vi "booleanvisibility.vi"() -> ()   [LabVIEW 2018]
panel:
  in  "stop 3":bool
  in  "String 2":string
  out "Numeric":i32
  in  "Boolean":bool
  in  "stop 2":bool
  in  "String":string
  in  "Boolean 2":bool
  in  "stop":bool
  in  "visible":bool
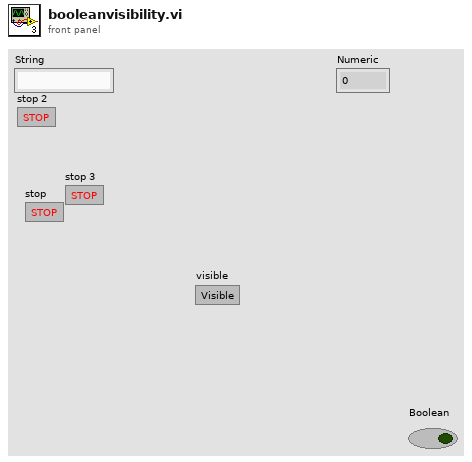
[diagram p1: front panel]
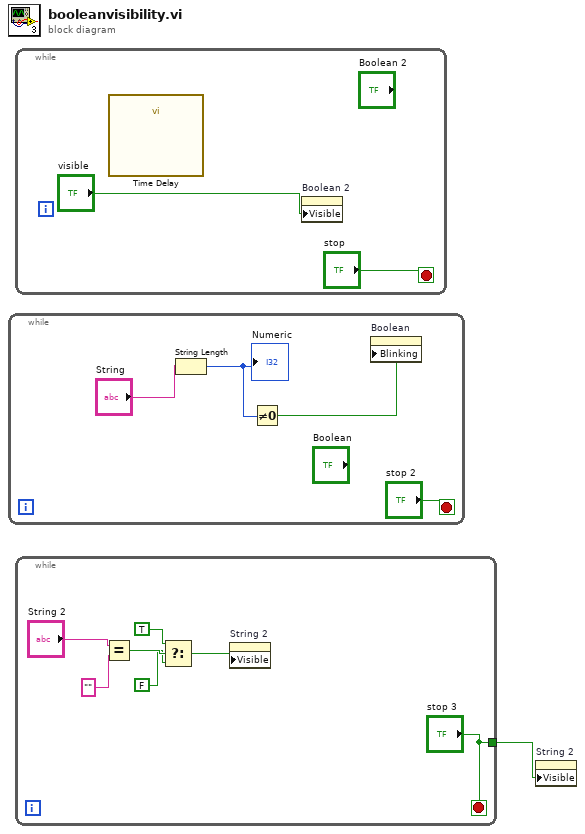
[diagram p0: block diagram]
diagram:
  n1 = while {
    stop <- "stop 2" stop-if-true
    n2 = String Length(string="String") -> (length=w3:i32)
    "Numeric" <- w3
    n3 = Not Equal To 0?(x=w3) -> (x != 0?=w2:bool)
    n4 = property on="Boolean" class="Bool (strict)"("Blinking"=w2) -> ()  [unwired: 2 in, 2 out]
  }
  n5 = while {
    stop <- "stop" stop-if-true
    n6 = call "Time Delay"() -> ()  [unwired: 11 in, 1 out]
    n7 = property on="Boolean 2" class="Bool (strict)"("Visible"="visible") -> ()  [unwired: 2 in, 2 out]
  }
  n8 = while {
    tunnel: ["stop 3"] -> w1
    stop <- "stop 3" stop-if-true
    n9 = Equal?(x="String 2", y="") -> (x = y?=w12:bool)
    n10 = Select(t=TRUE, s=w12, f=FALSE) -> (s? t:f=w9:bool)
    n11 = property on="String 2" class="Str"("Visible"=w9) -> ()  [unwired: 2 in, 2 out]
  }
  n12 = property on="String 2" class="Str"("Visible"=w1) -> ()  [unwired: 2 in, 2 out]
